vi "DSF.Shared.Configuration.Transfer Group.Check.Transfers.vi"(8 "error in (no error)":errorcluster, 10 "Transfer Configurations in":refnum<class "DSF.Shared.Configuration.Transfer.lvclass">[](array[class]), 11 "Transfer Group Configuration in":refnum<class "DSF.Shared.Configuration.Transfer Group.lvclass">) -> (0 "error out":errorcluster, 2 "Transfer Configurations out":refnum<class "DSF.Shared.Configuration.Transfer.lvclass">[](array[class]), 3 "Transfer Group Configuration out":refnum<class "DSF.Shared.Configuration.Transfer Group.lvclass">)   [LabVIEW 2016, in "DSF.Shared.lvlib" / "DSF.Shared.Configuration.Transfer Group.lvclass"]
uses:
  DSF.Shared.Configuration.Transfer Group.lvclass
  Transfer/DSF.Shared.Configuration.Transfer.lvclass
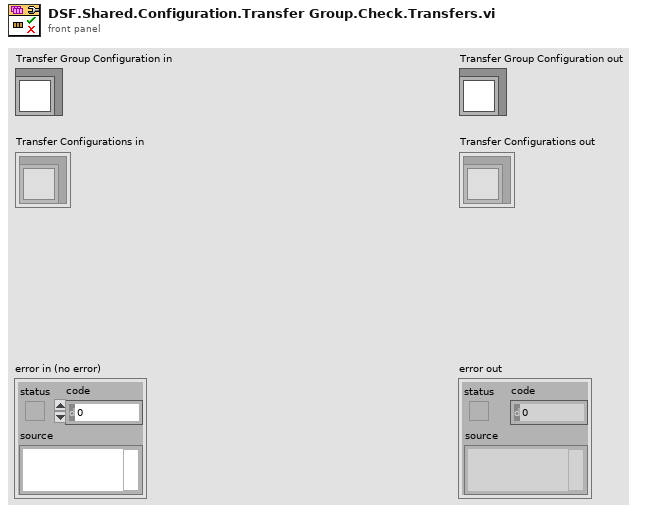
[diagram p1: front panel]
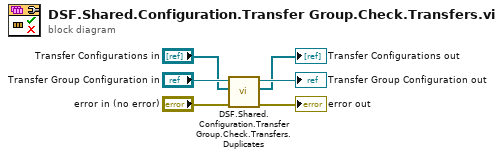
[diagram p0: block diagram]
diagram:
  n1 = call "DSF.Shared.Configuration.Transfer Group.Check.Transfers.Duplicates.vi"("error in (no error)"="error in (no error)", "Transfer Configurations in"="Transfer Configurations in", "Transfer Group Configuration in"="Transfer Group Configuration in") -> ("error out"=→"error out":errorcluster, "Transfer Configurations out"=→"Transfer Configurations out":refnum<class "DSF.Shared.Configuration.Transfer.lvclass">[], "Transfer Group Configuration out"=→"Transfer Group Configuration out":refnum<class "DSF.Shared.Configuration.Transfer Group.lvclass">)  [unwired: 6 in]
